vi "PDUsJasonToArray.vi"(8 "error in (no error)":errorcluster, 11 "Data Out":string) -> (0 "error out":errorcluster, 3 "PUIDs":string[](array[string]))   [LabVIEW 2015]
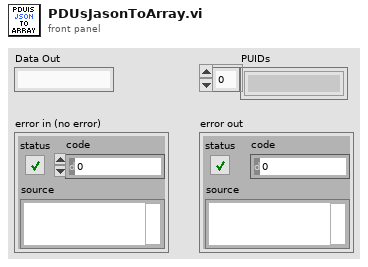
[diagram p1: front panel]
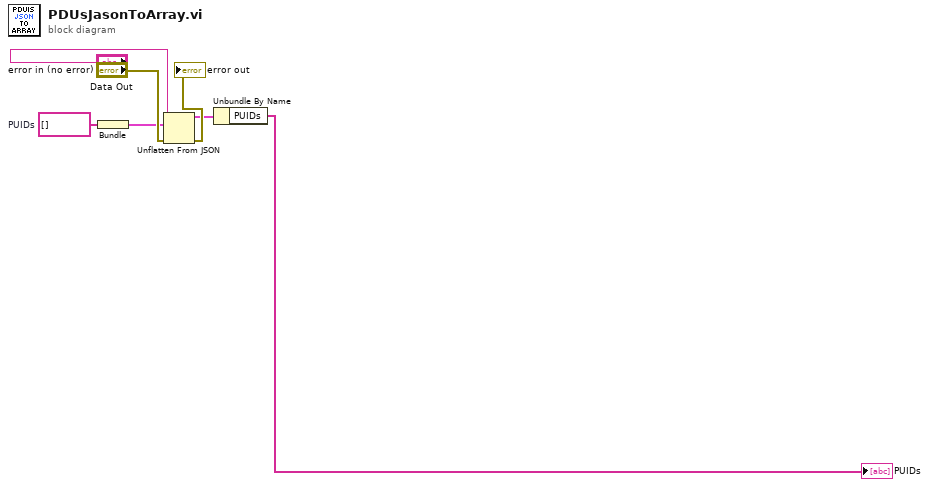
[diagram p0: block diagram]
diagram:
  w3 = string[] []  # PUIDs
  n1 = Bundle("PUIDs"=w3) -> (w2:cluster{"PUIDs":string[]})  [unwired: 1 in]
  n2 = Unflatten From JSON(JSON string="Data Out", type and defaults=w2, error in (no error)="error in (no error)") -> (value=w1:cluster{"PUIDs":string[]}, error out=→"error out":errorcluster)  [unwired: 4 in]
  n3 = Unbundle By Name(w1) -> ("PUIDs"=→"PUIDs":string[])
